vi "Sensorer 3 (SubVI).vi"(9 "ZERO ALL SENSORS":bool, 10 "Sensor 3 (A/AI2(Pin7))":dbl, 11 "Filtered x in":dbl) -> (1 "Filtered x out":dbl, 2 "F.L Rear Leftt":T1(graph), 3 "Sensor 1":dbl=0.0038137989155123176 format="%0.5f")   [LabVIEW 2019]
uses:
  <vilib>/ptbypt/NI_PtbyPt.lvlib
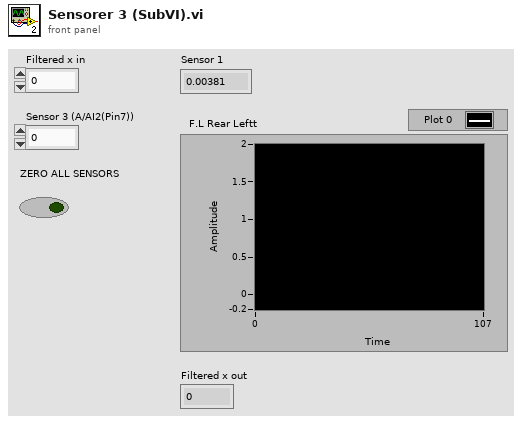
[diagram p1: front panel]
types:
  T1 = cluster{"Filtered x":dbl, "Sensor 1 (A/AI0 (Pin 3))":dbl}
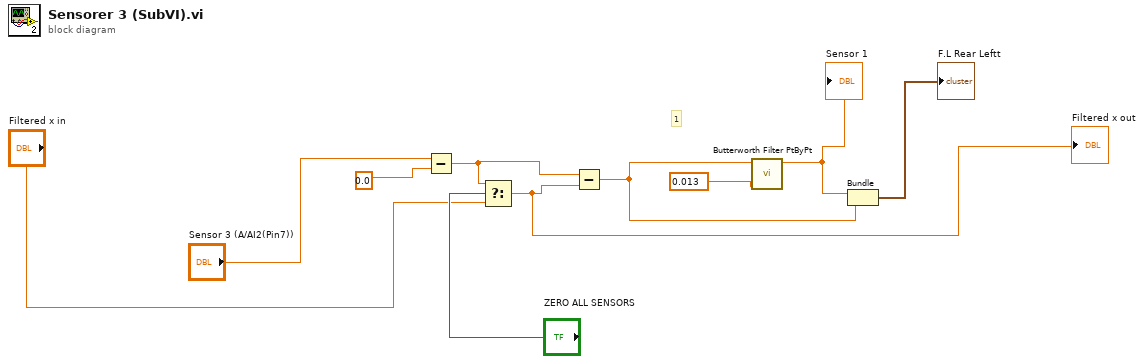
[diagram p0: block diagram]
diagram:
  # "1"
  n1 = Subtract(x="Sensor 3 (A/AI2(Pin7))", y=0.0) -> (x-y=w3:dbl)
  n2 = Select(t=w3, s="ZERO ALL SENSORS", f="Filtered x in") -> (s? t:f=w1:dbl)
  "Filtered x out" <- w1
  n3 = Subtract(x=w3, y=w1) -> (x-y=w7:dbl)
  n4 = call <vilib>:"Butterworth Filter PtByPt.vi"("low cutoff freq: fl"=0.013 ("low cutoff freq: 1"), "x"=w7) -> ("Filtered x"=w10:dbl)  [unwired: 7 in, 1 out]
  "Sensor 1" <- w10
  n5 = Bundle("Filtered x"=w10, w7) -> (→"F.L Rear Leftt":cluster{"Filtered x":dbl, dbl})  [unwired: 1 in]
